vi "Password-File-Path.vi"() -> (3 "Matched Config File":path)   [LabVIEW 2020]
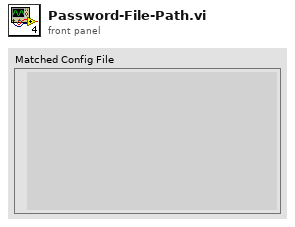
[diagram p1: front panel]
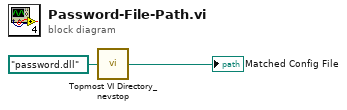
[diagram p0: block diagram]
diagram:
  n1 = call <userlib>:"Topmost VI Directory_nevstop.vi"("Relative path (.)"=path "password.dll") -> ("Application Directory (+ Relative)"=→"Matched Config File":path)  [unwired: 4 in]
